vi "Revision Query.vi"(8 "error in (no error)":errorcluster, 11 "VISA resource name":refnum<visa-resource-name>) -> (0 "error out":errorcluster, 1 "Instrument Firmware Revision":string, 2 "Instrument Driver Revision":string, 3 "VISA resource name out":refnum<visa-resource-name>)   [LabVIEW 2018, in "JULABO DeviceDriver.lvlib"]
doc: "Queries the current instrument firmware revision and instrument driver revision.\n\nRefer to the Readme file for detailed driver information including modification history."
uses:
  JULABO DeviceDriver.lvlib
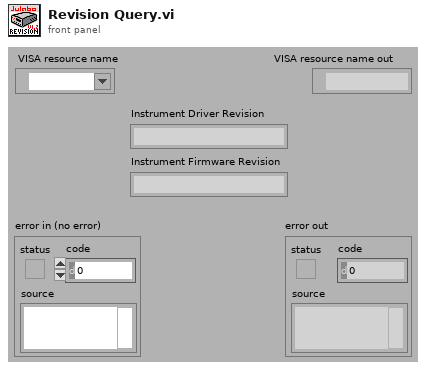
[diagram p1: front panel]
types:
  T1 = cluster{"Major":u16, "Minor":u16, "Fix":u16, "Build":u16}
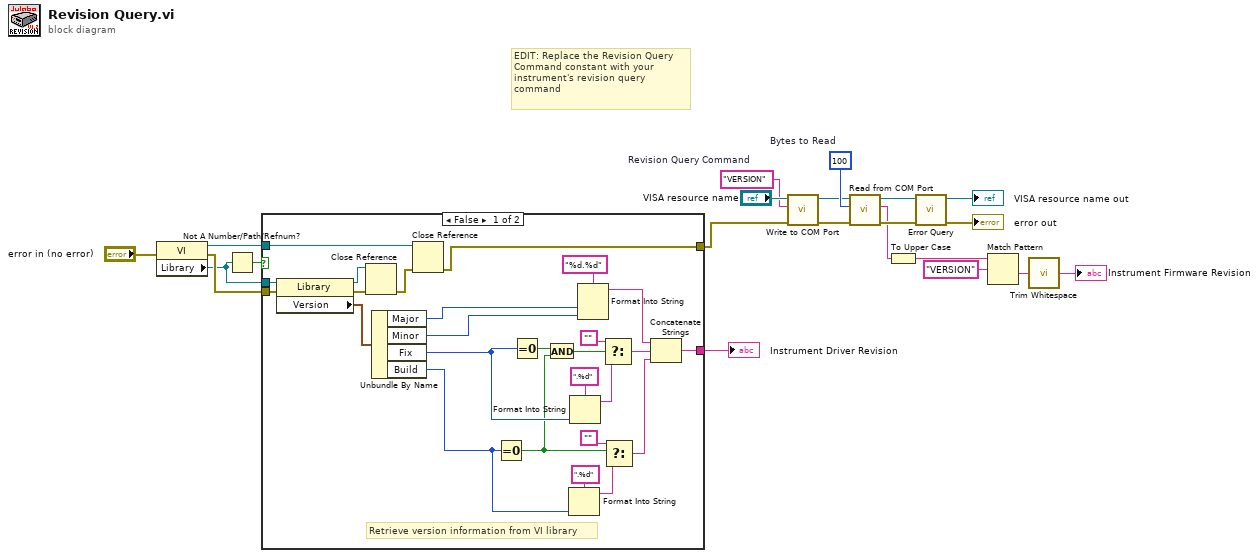
[diagram p0: block diagram]
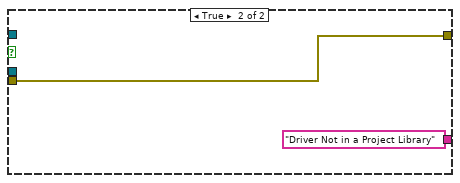
[diagram p2: hidden frame]
diagram:
  w17 = "VERSION"  # Revision Query Command
  w20 = u32 100  # Bytes to Read
  # "EDIT: Replace the Revision Query\nCommand constant with your\ninstrument's revision query\ncommand"
  n1 = property class="VI"(error in="error in (no error)") -> (reference out=w12:refnum<vi>, error out=w11:errorcluster, "Library"=w10:refnum<vi>)  [unwired: 1 in]
  n2 = Not A Number/Path/Refnum?(number/path/refnum=w10) -> (NaN/Path/Refnum?=w9:bool)
  n3 = case shown="False" w9 {
    tunnel: w12 -> [w44 _]
    tunnel: w11 -> [w29 w49]
    tunnel: [w24 w49] -> w6
    tunnel: [w23 "Driver Not in a Project Library"] -> w8
    tunnel: w10 -> [w22 _]
    frame False {
      # "Retrieve version information from VI library"
      n4 = property class="Library"(reference=w22, error in=w29) -> (reference out=w46:refnum<vi>, error out=w47:errorcluster, "Version"=w43:T1)
      n5 = Close Reference(reference=w46, error in (no error)=w47) -> (error out=w45:errorcluster)
      n6 = Unbundle By Name(w43) -> ("Major"=w32:u16, "Minor"=w31:u16, "Fix"=w28:u16, "Build"=w30:u16)
      n7 = Close Reference(reference=w44, error in (no error)=w45) -> (error out=w24:errorcluster)
      n8 = Equal To 0?(x=w30) -> (x = 0?=w26:bool)
      n9 = Equal To 0?(x=w28) -> (x = 0?=w27:bool)
      n10 = And(x=w27, y=w26) -> (x .and. y?=w25:bool)
      n11 = Format Into String(format string=".%d", w30) -> (resulting string=w36:string)  [unwired: 2 in, 1 out]
      n12 = Format Into String(format string=".%d", w28) -> (resulting string=w40:string)  [unwired: 2 in, 1 out]
      n13 = Format Into String(format string="%d.%d", w32, w31) -> (resulting string=w38:string)  [unwired: 2 in, 1 out]
      n14 = Select(t="", s=w25, f=w40) -> (s? t:f=w37:string)
      n15 = Select(t="", s=w26, f=w36) -> (s? t:f=w33:string)
      n16 = Concatenate Strings(w38, w37, w33) -> (w23:string)
    }
    frame True {
    }
  }
  "Instrument Driver Revision" <- w8
  n17 = call "Write to COM Port.vi"("error in"=w6, "Command (input)"=w17, "VISA resource name in"="VISA resource name") -> ("error out"=w18:errorcluster, "VISA resource name out"=w19:refnum<visa-resource-name>)  [unwired: 7 in]
  n18 = call "Read from COM Port.vi"("error in"=w18, "Byte to Read (-1:All)"=w20, "VISA resource name in"=w19) -> ("error out"=w16:errorcluster, "String (output)"=w5:string, "VISA resource name out"=w15:refnum<visa-resource-name>)  [unwired: 5 in, 1 out]
  n19 = To Upper Case(1:w5) -> (0:w1:string)
  n20 = call "Error Query.vi"("error in (no error)"=w16, "VISA resource name"=w15) -> ("error out"=→"error out":errorcluster, "VISA resource name out"=→"VISA resource name out":refnum<visa-resource-name>)  [unwired: 6 in, 2 out]
  n21 = Match Pattern(string=w1, regular expression="VERSION" ("regulärer Ausdruck")) -> (after substring=w3:string)  [unwired: 1 in, 3 out]
  n22 = call <vilib>:"Trim Whitespace.vi"("string"=w3) -> ("trimmed string"=→"Instrument Firmware Revision":string)  [unwired: 1 in]
